vi "Scan IM 120 x 80 Test Panel.vi"() -> ()   [LabVIEW 2020]
uses:
  <userlib>/Tango_DLL/Tango_DLL.lvlib
panel:
  out "Position":dbl[](array[numeric])
  out "Waiting for Reply":bool
  out "Last Error":errorcluster
  out "Command History":string
  out "Reply":string
  in  "Command":string
  in  "Quit":bool
  in  "COM Port":refnum<visa-resource-name>="COM4"
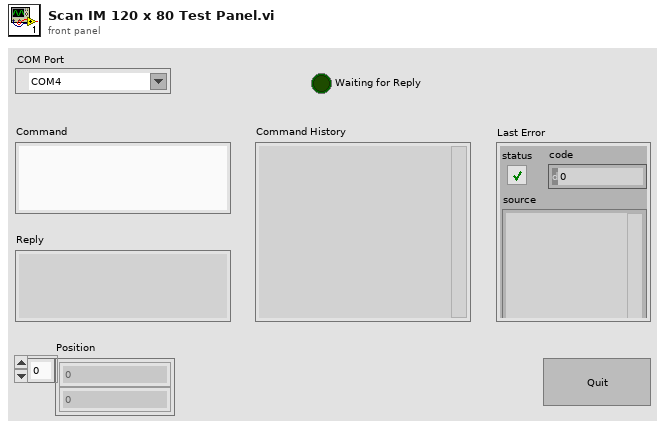
[diagram p1: front panel]
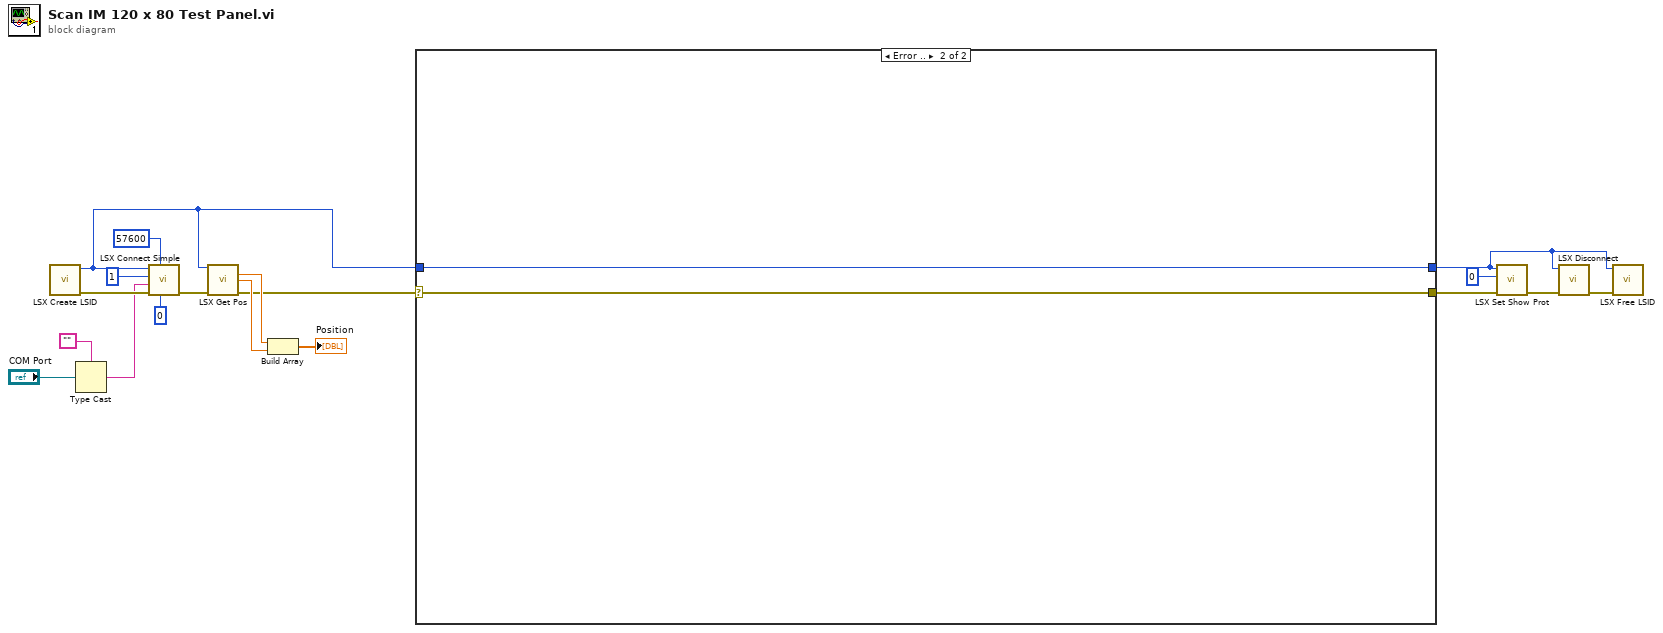
[diagram p0: block diagram]
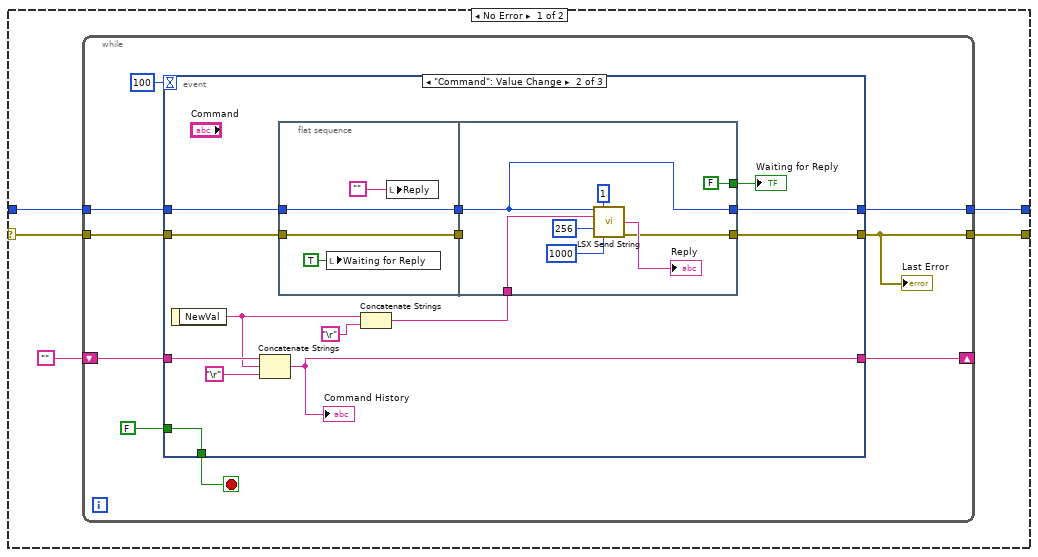
[diagram p2: hidden frame]
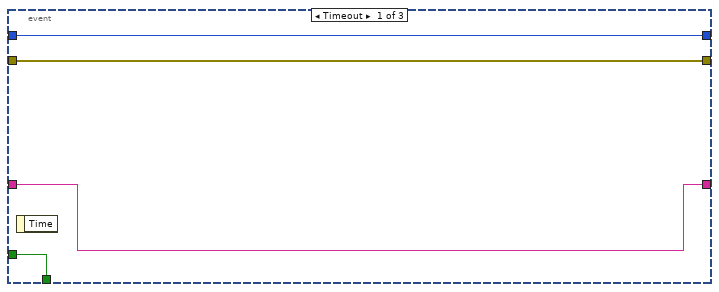
[diagram p3: hidden frame]
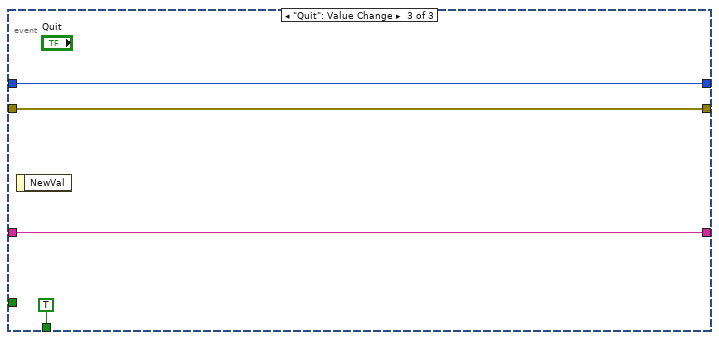
[diagram p4: hidden frame]
diagram:
  n1 = call <userlib>:"LSX Create LSID.vi"() -> ("error out"=w18:errorcluster, "plLSID out"=w9:i32)  [unwired: 9 in, 1 out]
  n2 = Type Cast(type="", x="COM Port") -> (*(type *) &x=w6:string)
  n3 = call <userlib>:"LSX Connect Simple.vi"("bAShowProt"=0, "lABaudRate"=57600, "error in (no error)"=w18, "pcAComName"=w6, "lAnInterfaceType"=1, "lLSID"=w9) -> ("error out"=w14:errorcluster)  [unwired: 3 in, 2 out]
  n4 = call <userlib>:"LSX Get Pos.vi"("lLSID"=w9, "error in (no error)"=w14) -> ("pdX out"=w13:dbl, "pdY out"=w12:dbl, "error out"=w10:errorcluster)  [unwired: 8 in, 3 out]
  n5 = Build Array(w13, w12) -> (→"Position":dbl[])
  n6 = case shown="Error .." w10 {
    selector: w10 -> [w22 w67]
    tunnel: w9 -> [w23 w68]
    tunnel: [w21 w68] -> w2
    tunnel: [w20 w67] -> w1
    frame No Error {
      n7 = while {
        tunnel: w23 -> [w30]
        tunnel: w22 -> [w29]
        tunnel: [w28] -> w21
        tunnel: [w25] -> w20
        shift-right: [w26] -> _
        shift-left: "" -> [w27]
        stop <- w31 stop-if-true
        n8 = event shown="[1] \"Command\": Value Change" {
          selector: _ -> [_ _ _]
          dyn-events: _ -> [_ _ _]
          timeout: 100 -> [_ _ _]
          tunnel: FALSE -> [w36 w50 _]
          tunnel: [w36 w50 TRUE] -> w31
          tunnel: w30 -> [w34 w49 w63]
          tunnel: w29 -> [w33 w48 w66]
          tunnel: [w34 w40 w63] -> w28
          tunnel: [w33 w45 w66] -> w25
          tunnel: w27 -> [w35 w43 w64]
          tunnel: [w35 w42 w64] -> w26
          event Timeout {
            n9 = event-data() -> ()  [unwired: 1 in, 1 out]
          }
          event "Command": Value Change {
            n10 = event-data() -> ("NewVal"=w39:string)  [unwired: 1 in]
            n11 = Concatenate Strings(w43, w39, "\r") -> (w42:string)
            "Command History" <- w42
            n12 = flat-sequence {
              tunnel: w48 -> [w53]
              tunnel: w49 -> [w54]
              tunnel: [w54] -> w47
              tunnel: [w53] -> w46
              tunnel: w47 -> [w56]
              tunnel: w46 -> [_]
              tunnel: [w57] -> w45
              tunnel: [FALSE] -> w41
              tunnel: [w56] -> w40
              tunnel: w38 -> [w55]
              frame #0 {
                n13 = local write "Waiting for Reply"(TRUE ("Waiting for Cmd")) -> ()
                n14 = local write "Reply"("") -> ()
              }
              frame #1 {
                n15 = call <userlib>:"LSX Send String.vi"("lLSID"=w56, "bReadLine"=1, "pcStr"=w55, "lMaxLen"=256, "lTimeOut"=1000) -> ("pcRet out"=→"Reply":string, "error out"=w57:errorcluster)  [unwired: 7 in, 2 out]
              }
            }
            n16 = Concatenate Strings(w39, "\r") -> (w38:string)
            "Waiting for Reply" <- w41
          }
          event "Quit": Value Change {
            n17 = event-data() -> ()  [unwired: 1 in, 1 out]
          }
        }
        "Last Error" <- w25
      }
    }
    frame Error {
    }
  }
  n18 = call <userlib>:"LSX Set Show Prot.vi"("error in (no error)"=w1, "bShowProt"=0, "lLSID"=w2) -> ("error out"=w4:errorcluster)  [unwired: 7 in, 1 out]
  n19 = call <userlib>:"LSX Disconnect.vi"("error in (no error)"=w4, "lLSID"=w2) -> ("error out"=w5:errorcluster)  [unwired: 8 in, 1 out]
  n20 = call <userlib>:"LSX Free LSID.vi"("error in (no error)"=w5, "lLSID"=w2) -> ()  [unwired: 8 in, 2 out]
